vi "Update Sensor Info and Re-broadcast.vi"(8 "error in (no error)":errorcluster, 10 "SensorInfo":refnum<class "SensorInfo.lvclass">, 11 "Sensor in":refnum<class "Sensor.lvclass">) -> (0 "error out":errorcluster, 3 "Sensor out":refnum<class "Sensor.lvclass">)   [LabVIEW 2012, in "Sensor Definition.lvlib" / "Sensor.lvclass"]
uses:
  Sensor.lvclass
  SensorInfo.lvclass
  Sensor.lvclass/Sensor.ctl
  SensorInfo.lvclass/SensorInfo.ctl
  SensorInfo/Read Sample Time.vi
  Read SensorInfo.vi
  Write SensorInfo.vi
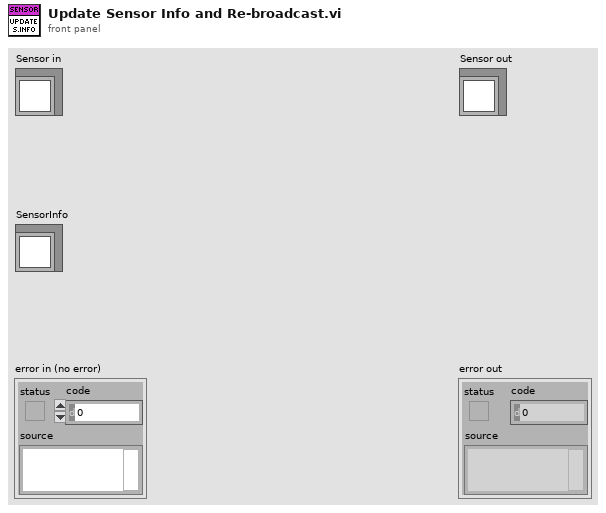
[diagram p1: front panel]
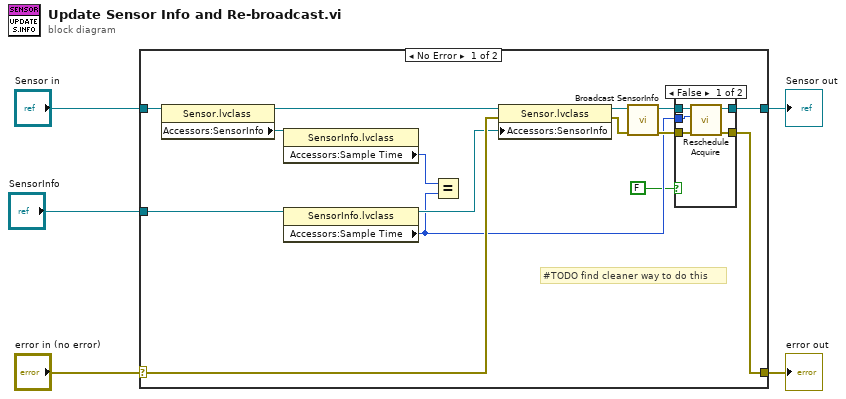
[diagram p0: block diagram]
diagram:
  n1 = case shown="No Error" "error in (no error)" {
    selector: "error in (no error)" -> [w19 w29]
    tunnel: [w8 w29] -> w4
    tunnel: [w10 w28] -> w2
    tunnel: "Sensor in" -> [w20 w28]
    tunnel: "SensorInfo" -> [w14 _]
    frame No Error {
      # "#TODO find cleaner way to do this"
      n2 = property class="Sensor.lvclass"(reference=w20) -> (reference out=w16:refnum<class "Sensor.lvclass">, "Accessors:SensorInfo"=w15:refnum<class "SensorInfo.lvclass">)  [unwired: 1 in, 1 out]
      n3 = property class="SensorInfo.lvclass"(reference=w15) -> ("Accessors:Sample Time"=w12:i32)  [unwired: 1 in, 2 out]
      n4 = property class="SensorInfo.lvclass"(reference=w14) -> (reference out=w13:refnum<class "SensorInfo.lvclass">, "Accessors:Sample Time"=w7:i32)  [unwired: 1 in, 1 out]
      n5 = Equal?(x=w12, y=w7) -> ()  [unwired: 1 out]
      n6 = property class="Sensor.lvclass"(reference=w16, error in=w19, "Accessors:SensorInfo"=w13) -> (reference out=w18:refnum<class "Sensor.lvclass">, error out=w17:errorcluster)
      n7 = call "Broadcast SensorInfo.vi"("error in (no error)"=w17, "Sensor in"=w18) -> ("error out"=w9:errorcluster, "Sensor out"=w11:refnum<class "Sensor.lvclass">)  [unwired: 8 in]
      n8 = case shown="False" FALSE {
        tunnel: w11 -> [w25 w27]
        tunnel: [w24 w27] -> w10
        tunnel: w9 -> [w23 w26]
        tunnel: [w22 w26] -> w8
        tunnel: w7 -> [w21 _]
        frame False {
          n9 = call-dynamic "Reschedule Acquire.vi"("error in (no error)"=w23, "Sample Time"=w21, "Sensor in"=w25) -> ("error out"=w22:errorcluster, "Sensor out"=w24:refnum<class "Sensor.lvclass">)  [unwired: 7 in]
        }
        frame True {
        }
      }
    }
    frame Error {
    }
  }
  "error out" <- w4
  "Sensor out" <- w2
